vi "Construct Queue Transport.vi"(10 "Max Queue Size (-1)":i32=-1) -> (0 "error out":errorcluster, 3 "QueueTransport":refnum<class "QueueTransport.lvclass">)   [LabVIEW 2018, in "MVA Framework.lvlib" / "QueueTransport.lvclass"]
doc: "构建队列传输"
uses:
  QueueTransport.lvclass
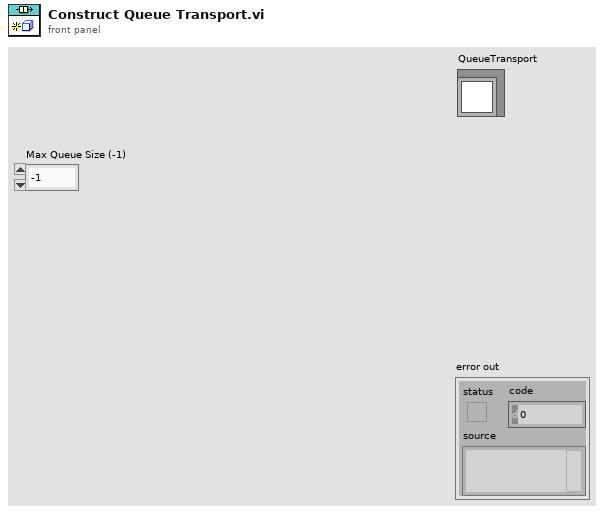
[diagram p1: front panel]
types:
  T1 = cluster{"Data":variant, "Publication Time":timestamp}
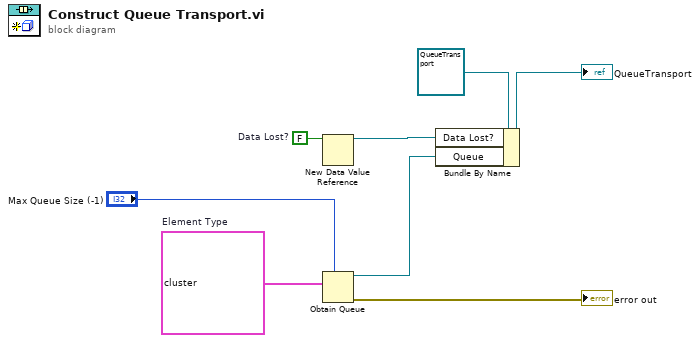
[diagram p0: block diagram]
diagram:
  w2 = FALSE  # Data Lost?
  w5 = T1 {"Data"=variant, "Publication Time"=timestamp(0 s since 1904-01-01)}  # Element Type
  n1 = New Data Value Reference(data value=w2) -> (data value reference=w1:refnum<data-value>)  [unwired: 1 in, 1 out]
  n2 = Obtain Queue(max queue size (-1, unlimited)="Max Queue Size (-1)", element data type=w5) -> (queue out=w4:refnum<queue>, error out=→"error out":errorcluster)  [unwired: 3 in, 1 out]
  n3 = Bundle By Name(cluster=refnum<class "QueueTransport.lvclass"> refnum ("QueueTransport.lvclass"), "Data Lost?"=w1, "Queue"=w4) -> (→"QueueTransport":refnum<class "QueueTransport.lvclass">)
